vi "Render Ship Strings.vi"(6 "Player":T1, 8 "error in (no error)":errorcluster, 11 "Main Controller Actor in":refnum<class "Main Controller Actor.lvclass">) -> (0 "error out":errorcluster)   [LabVIEW 2021, in "Main Controller Actor.lvclass"]
uses:
  Main Controller Actor.lvclass
  Player.ctl
  Ship/Ship.lvclass
  Main Controller Actor.lvclass/Main Controller Actor.ctl
  Ship/Ship.lvclass/Ship.ctl
  Re-use Libraries/Vector 2D/Vector 2D.lvclass/Vector 2D.ctl
  Sprite Font/Sprite Font.lvclass
  Re-use Libraries/Vector 2D/Vector 2D.lvclass
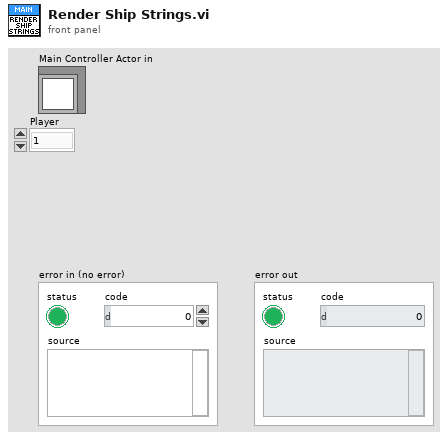
[diagram p1: front panel]
types:
  T1 = typedef "Main Controller Actor.lvclass/Player.ctl" = enum16{"1", "2"}
  T2 = typedef "Constants.ctl" = cluster{"Colours":cluster{"OK":u32, "Warning":u32, "Error":u32, "Red":u32, "Green":u32, "Blue":u32, "Yellow":u32}, "System":cluster{"Target Frames Second":dbl, "World Size":T3, "Window Size":T3, "Battle Area Size":T3, "Sidebar Width":sgl, "SC2 Frame Rate [Seconds/Frame]":sgl, "Sidebar Player 2 Y Offset":sgl, "Windows Size V2":refnum<class "Vector 2D.lvclass">, "World Size V2":refnum<class "Vector 2D.lvclass">, "Battle Area Size V2":refnum<class "Vector 2D.lvclass">}, "Game":cluster{"Maximum Asteroids":i32, "Max Energy":i32, "Max Crew":i32, "Maximum Stars":i32}}
  T3 = typedef "SDL2 Utility.lvlib/Point (I32).ctl" = cluster{"x":i32, "y":i32}
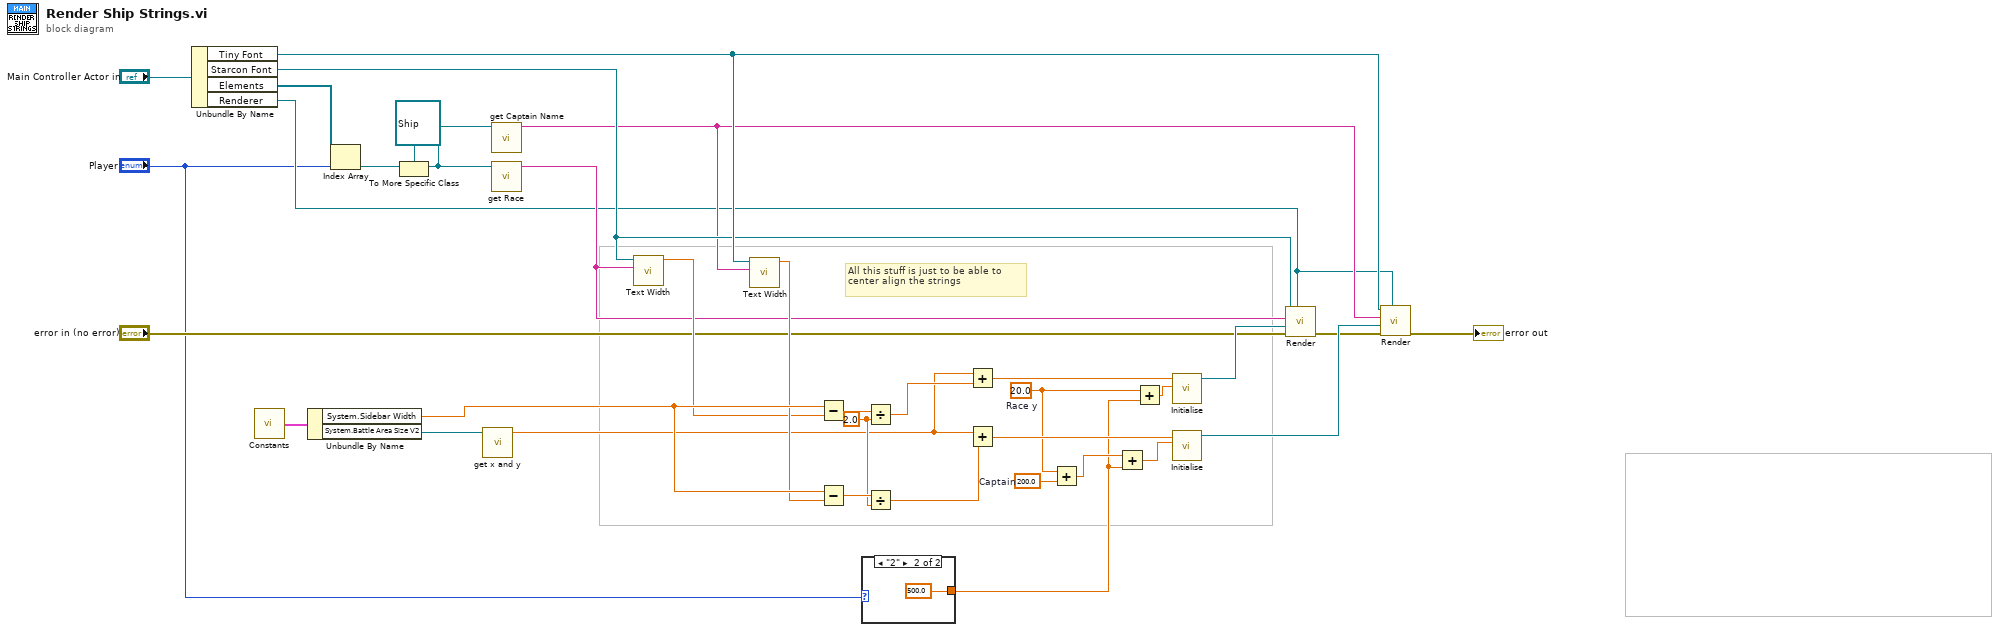
[diagram p0: block diagram]
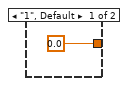
[diagram p2: hidden frame]
diagram:
  w12 = sgl 200.0  # Captain
  w3 = sgl 2.0 ("y")
  w9 = sgl 20.0  # Race y
  # "All this stuff is just to be able to center align the strings"
  n1 = Unbundle By Name("Main Controller Actor in") -> ("Tiny Font"=w33:refnum<class "Sprite Font.lvclass">, "Starcon Font"=w32:refnum<class "Sprite Font.lvclass">, "Elements"=w16:refnum<class "Element.lvclass">[], "Renderer"=w13:refnum<class "Renderer.lvclass">)
  n2 = call "Constants.vi"() -> ("Constants"=w34:T2)
  n3 = Unbundle By Name(w34) -> ("System.Sidebar Width"=w35:sgl, "System.Battle Area Size V2"=w2:refnum<class "Vector 2D.lvclass">)
  n4 = Index Array(array=w16, index="Player") -> (element=w17:refnum<class "Element.lvclass">)
  n5 = To More Specific Class(target class=refnum<class "Ship.lvclass"> refnum ("Ship.lvclass"), reference=w17) -> (specific class reference=w20:refnum<class "Ship.lvclass">)  [unwired: 1 in, 1 out]
  n6 = call "get x and y.vi"("Vector 2D in"=w2) -> ("x"=w1:sgl)  [unwired: 9 in, 1 out]
  n7 = call "get Captain Name.vi"("Ship in"=w20) -> ("Captain Name"=w27:string)  [unwired: 10 in]
  n8 = call "get Race.vi"("Ship in"=w20) -> ("Race"=w22:string)  [unwired: 10 in]
  n9 = call-dynamic "Text Width.vi"("String"=w22, "Font in"=w32) -> ("Width"=w23:sgl)  [unwired: 9 in]
  n10 = call-dynamic "Text Width.vi"("String"=w27, "Font in"=w33) -> ("Width"=w28:sgl)  [unwired: 9 in]
  n11 = Subtract(x=w35, y=w23) -> (x-y=w24:sgl)
  n12 = Subtract(x=w35, y=w28) -> (x-y=w30:sgl)
  n13 = case shown="\"2\"" "Player" {
    tunnel: [sgl 0.0 ("y") sgl 500.0 ("y")] -> w4
    frame "1", Default {
    }
    frame "2" {
    }
  }
  n14 = Divide(x=w24, y=w3) -> (x/y=w25:sgl)
  n15 = Divide(x=w30, y=w3) -> (x/y=w31:sgl)
  n16 = Add(x=w1, y=w25) -> (x+y=w26:sgl)
  n17 = Add(x=w1, y=w31) -> (x+y=w29:sgl)
  n18 = Add(x=w9, y=w12) -> (x+y=w7:sgl)
  n19 = Add(x=w7, y=w4) -> (x+y=w6:sgl)
  n20 = Add(x=w9, y=w4) -> (x+y=w8:sgl)
  n21 = call "Initialise.vi"("y"=w8, "x"=w26) -> ("Vector 2D out"=w19:refnum<class "Vector 2D.lvclass">)  [unwired: 9 in]
  n22 = call "Initialise.vi"("y"=w6, "x"=w29) -> ("Vector 2D out"=w21:refnum<class "Vector 2D.lvclass">)  [unwired: 9 in]
  n23 = call-dynamic "Render.vi"("Renderer"=w13, "error in (no error)"="error in (no error)", "Position"=w19, "String"=w22, "Font in"=w32) -> ("error out"=w11:errorcluster)  [unwired: 6 in]
  n24 = call-dynamic "Render.vi"("Renderer"=w13, "error in (no error)"=w11, "Position"=w21, "String"=w27, "Font in"=w33) -> ("error out"=→"error out":errorcluster)  [unwired: 6 in]
